vi "Variant Attributes to Section.vi"(8 "error in (no error)":errorcluster, 9 "Parameters":variant, 10 "Section":string, 11 "Refnum in":T1) -> (0 "error out":errorcluster, 3 "Refnum out":T1)   [LabVIEW 2009, in "POLARIS Vision utility.lvlib"]
uses:
  POLARIS Vision utility.lvlib
  <vilib>/Utility/config.llb/Config Data RefNum.ctl
  <vilib>/Utility/config.llb/Write Key (String).vi
  <vilib>/Utility/config.llb/Write Key (I32).vi
  <vilib>/Utility/config.llb/NI_LVConfig.lvlib
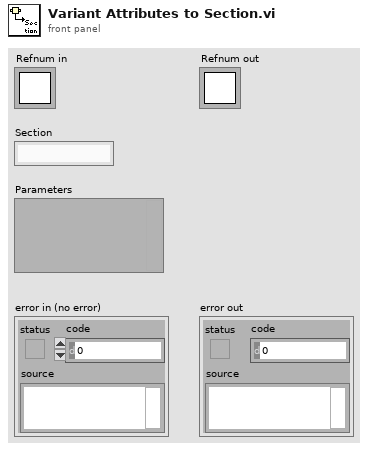
[diagram p1: front panel]
types:
  T1 = typedef "NI_LVConfig.lvlib/Config Data RefNum.ctl" = refnum<k1>
  T2 = typedef "Type Descriptor Enumeration__ogtk.ctl" = enum8{"<Null>", "I8", "I16", "I32", "I64", "U8", "U16", "U32", "U64", "SGL", "DBL", "EXT", "CSG", "CDB", "CXT", "0x0F", "0x10", "0x11", "0x12", "0x13", "0x14", "Enum U8", "Enum U16", "Enum U32", "Enum U64", "SGL PQ", "DBL PQ", "EXT PQ", "CSG PQ", "CDB PQ", "CXT PQ", "0x1F", "0x20", "Boolean", "0x22", "0x23", "0x24", "0x25", "0x26", "0x27", "0x28", "0x29", "0x2A", "0x2B", "0x2C", "0x2D", "0x2E", "0x2F", "String", "0x31", "Path", "Pict", "0x34", "0x35", "0x36", "DAQ", "0x38", "0x39", "0x3A", "0x3B", "0x3C", "0x3D", "0x3E", "0x3F", "Array", "0x41", "0x42", "0x43", "0x44", "0x45", "0x46", "0x47", "0x48", "0x49", "0x4A", "0x4B", "0x4C", "0x4D", "0x4E", "0x4F", "Cluster", "0x51", "0x52", "Variant", "Waveform", "0x55", "0x56", "0x57", "0x58", "0x59", "0x5A", "0x5B", "0x5C", "0x5D", "0x5E", "0x5F", "0x60", "0x61", "0x62", "0x63", "0x64", "0x65", "0x66", "0x67", "0x68", "0x69", "0x6A", "0x6B", "0x6C", "0x6D", "0x6E", "0x6F", "Refnum"}
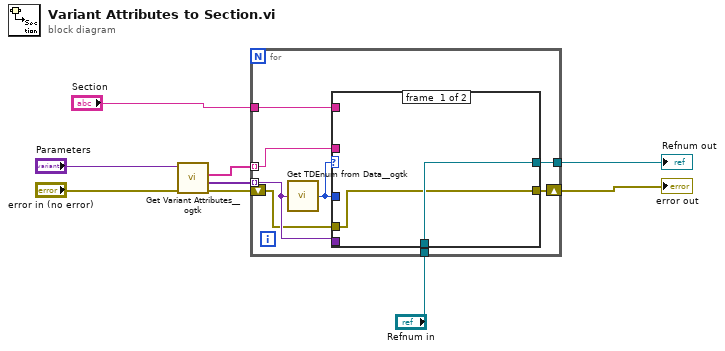
[diagram p0: block diagram]
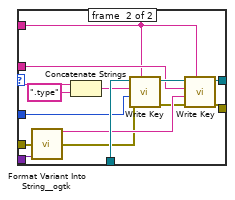
[diagram p2: hidden frame]
diagram:
  n1 = call "Get Variant Attributes__ogtk.vi"("error in"="error in (no error)", "Variant"="Parameters") -> ("error out"=w8:errorcluster, "value(s)"=w3:variant[], "names"=w4:string[])  [unwired: 2 in, 1 out]
  n2 = for {
    tunnel: w3 -> [w13] mode=indexing
    tunnel: w4 -> [w15] mode=indexing
    tunnel: "Refnum in" -> [w16]
    tunnel: [w17] -> w6
    tunnel: "Section" -> [w14]
    shift-right: [w12] -> w9
    shift-left: w8 -> [w11]
    n3 = call "Get TDEnum from Data__ogtk.vi"("Data"=w13) -> ("Type Descriptor Enumeration"=w10:T2)  [unwired: 4 in]
    n4 = case shown="Default" w10 {
      tunnel: [w19 w33] -> w17
      tunnel: w16 -> [w19 w32]
      tunnel: w15 -> [_ w30]
      tunnel: w14 -> [_ w27]
      tunnel: w10 -> [_ w26]
      tunnel: w13 -> [_ w25]
      tunnel: [w18 w22] -> w12
      tunnel: w11 -> [w18 w21]
      frame #0 {
      }
      frame #1 {
        n5 = call "Format Variant Into String__ogtk.vi"("error in (no error)"=w21, "Variant"=w25) -> ("Output String"=w24:string, "error out"=w20:errorcluster)  [unwired: 12 in]
        n6 = Concatenate Strings(w30, ".type" ("string")) -> (w28:string)
        n7 = call-poly <vilib>:"Write Key.vi"("section"=w27, "error in (no error)"=w20, "value"=w26, "key"=w28, "refnum"=w32) -> ("error out"=w23:errorcluster, "refnum out"=w31:T1)  [unwired: 4 in, 1 out]
        n8 = call-poly <vilib>:"Write Key.vi"("section"=w27, "error in (no error)"=w23, "value"=w24, "key"=w30, "refnum"=w31) -> ("error out"=w22:errorcluster, "refnum out"=w33:T1)  [unwired: 4 in, 1 out]
      }
    }
  }
  "error out" <- w9
  "Refnum out" <- w6
